vi "Send path to matlab.vi"(8 "error in":errorcluster) -> (0 "error out":errorcluster)   [LabVIEW 2013]
uses:
  Global Variables/General Globals.vi
panel:
  out "Execution time (ms)":u32
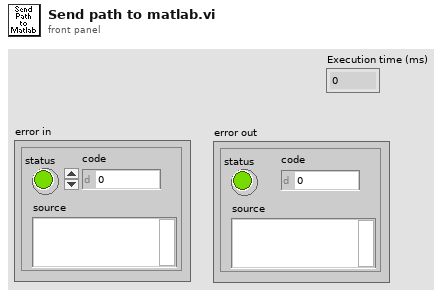
[diagram p1: front panel]
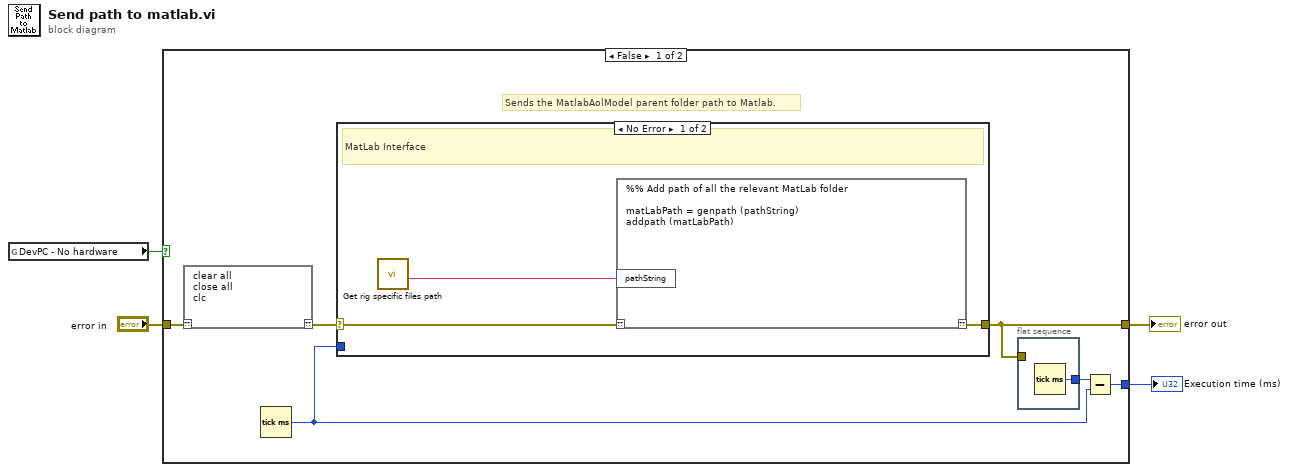
[diagram p0: block diagram]
diagram:
  n1 = global read "General Globals.vi" "DevPC - No hardware"() -> (w1:bool)
  n2 = case shown="False" w1 {
    tunnel: "error in" -> [w10 w16]
    tunnel: [w6 _] -> w3
    tunnel: [w5 w16] -> w2
    frame False {
      # "Sends the MatlabAolModel parent folder path to Matlab."
      n3 = script code="clear all\nclose all\nclc"("??"=w10) -> ("??"=w9:errorcluster)
      n4 = Tick Count (ms)() -> (millisecond timer value=w7:u32)
      n5 = case shown="No Error" w9 {
        selector: w9 -> [w14 w15]
        tunnel: [w13 w15] -> w5
        tunnel: w7 -> [_ _]
        frame No Error {
          # "MatLab Interface"
          n6 = call "Get rig specific files path.vi"() -> ("Rig-specific files folder (string)"=w12:string)  [unwired: 10 in, 1 out]
          n7 = script code="%% Add path of all the relevant MatLab folder\n\nmatLabPath = genpath (pathString)\naddpath (matLabPath)"("??"=w14, "pathString"=w12) -> ("??"=w13:errorcluster)
        }
        frame Error {
        }
      }
      n8 = flat-sequence {
        tunnel: [w11] -> w8
        tunnel: w5 -> [_]
        frame #0 {
          n9 = Tick Count (ms)() -> (millisecond timer value=w11:u32)
        }
      }
      n10 = Subtract(x=w8, y=w7) -> (x-y=w6:u32)
    }
    frame True {
      # "Demo mode / No hardware"
    }
  }
  "error out" <- w2
  "Execution time (ms)" <- w3
